vi "alternative instance of filter.vi"(7 "bandwidth":enum16{"20MHz", "40MHz"}(ring), 9 "input valid":bool, 10 "input cluster":T1) -> (1 "output valid":bool, 2 "sample out":T1)   [LabVIEW 2020]
uses:
  <vilib>/rvi/IPIntegrationNode/IPINode_Typedef/niFpgaIPINodeSupportedFamilies.ctl
  <vilib>/rvi/IPIntegrationNode/IPINode_Utilities/niFpgaIPINodeSimCore.vi
  <vilib>/rvi/XilinxIP/XIPIN_XNode/niFpgaXIPIN.xnode
  Untitled 3/FIR Compiler 3 1/xsim.dir/FIR_Compiler_3_1_CC812A82826341AB8BB5EFDFB4B49B09/xsimk_CC812A82826341AB8BB5EFDFB4B49B09.dll
  <vilib>/rvi/IPIntegrationNode/IPINode_Xnode/niFpgaIPINode.xnode
  Untitled 3/FIR Compiler 3 1 2/xsim.dir/FIR_Compiler_3_1_2_1438C8CDDF83493586378C164F746E96/xsimk_1438C8CDDF83493586378C164F746E96.dll
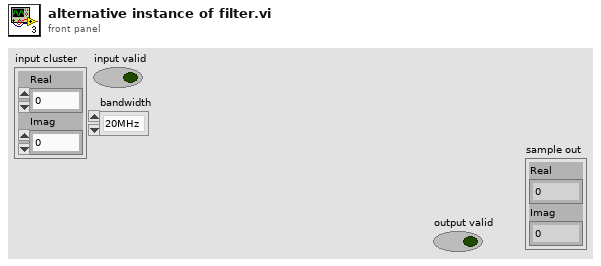
[diagram p1: front panel]
types:
  T1 = cluster{"Real":fxp<+/-,16,3>, "Imag":fxp<+/-,16,3>}
  T2 = typedef "niFpgaIPINodeSupportedFamilies.ctl" = cluster{"unlimited?":bool, "supported targets":string[]}
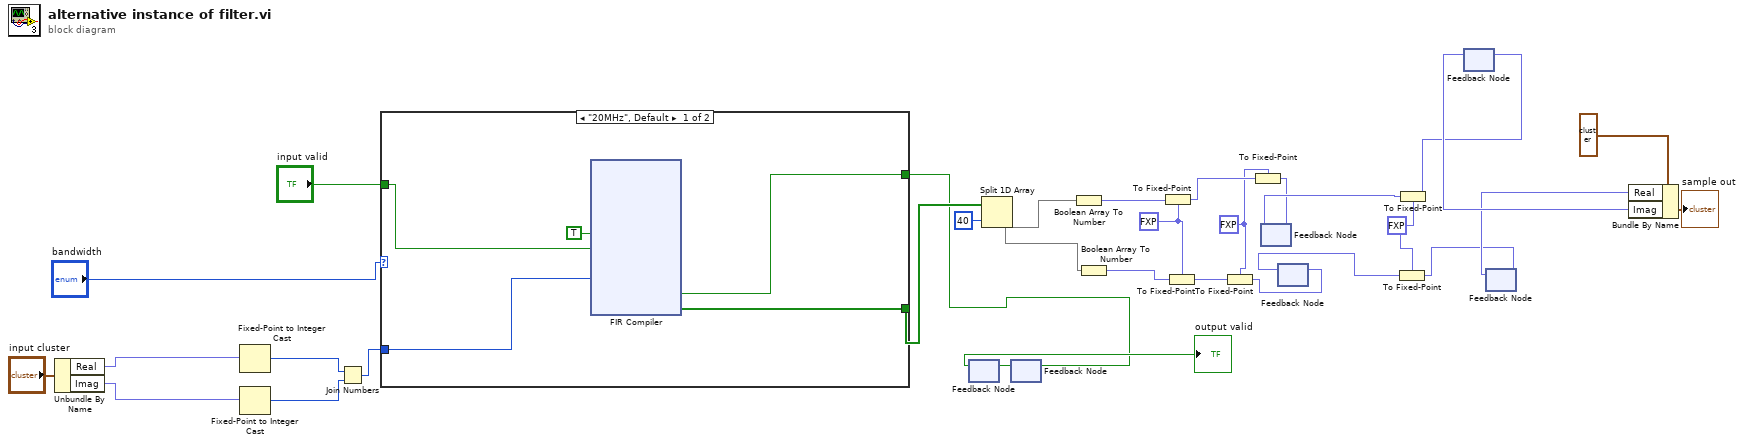
[diagram p0: block diagram]
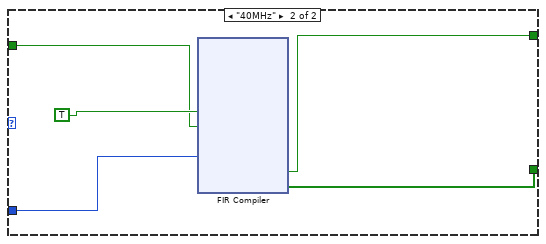
[diagram p2: hidden frame]
diagram:
  w10 = fxp<+/-,16,3> 0.0 ("fixed-point type")
  w9 = fxp<+/-,18,5> 0.0 ("fixed-point type")
  w8 = fxp<+/-,34,4> 0.0 ("fixed-point type")
  n1 = Unbundle By Name("input cluster") -> ("Real"=w12:fxp<+/-,16,3>, "Imag"=w13:fxp<+/-,16,3>)
  n2 = Fixed-Point to Integer Cast(1:w12) -> (0:w14:i16)
  n3 = Fixed-Point to Integer Cast(1:w13) -> (0:w15:i16)
  n4 = Join Numbers(hi=w14, lo=w15) -> ((hi.lo)=w17:u32)
  n5 = case shown="\"20MHz\", Default" "bandwidth" {
    tunnel: w17 -> [w37 w106]
    tunnel: [w36 w108] -> w30
    tunnel: [w35 w107] -> w1
    tunnel: "input valid" -> [w34 w104]
    frame "20MHz", Default {
      n6 = xnode ("FIR Compiler")("aclken"=TRUE, "s_axis_data_tvalid"=w34, "s_axis_data_tdata"=w37) -> ("m_axis_data_tvalid"=w35:bool, "m_axis_data_tdata"=w36:bool[])  [unwired: 1 out]
    }
    frame "40MHz" {
      n7 = xnode ("FIR Compiler")("aclken"=TRUE, "s_axis_data_tvalid"=w104, "s_axis_data_tdata"=w106) -> ("m_axis_data_tvalid"=w107:bool, "m_axis_data_tdata"=w108:bool[])  [unwired: 1 out]
    }
  }
  n8 = feedback #1() -> (→"output valid":bool)  [unwired: 1 in]
  n9 = Split 1D Array(array=w30, index=40) -> (first subarray=w19:bool[], second subarray=w20:bool[])
  n10 = feedback #2() -> (w2:bool)  [unwired: 1 in]
  n11 = feedback-in #1(w2) -> ()
  n12 = feedback-in #2(w1) -> ()
  n13 = Boolean Array To Number(Boolean array=w19) -> (number=w21:fxp<+/-,40,10>)
  n14 = Boolean Array To Number(Boolean array=w20) -> (number=w22:fxp<+/-,40,10>)
  n15 = To Fixed-Point(fixed-point type=w8, number=w21) -> (fixed-point=w23:fxp<+/-,34,4>)
  n16 = To Fixed-Point(fixed-point type=w8, number=w22) -> (fixed-point=w24:fxp<+/-,34,4>)
  n17 = To Fixed-Point(fixed-point type=w9, number=w24) -> (fixed-point=w4:fxp<+/-,18,5>)
  n18 = To Fixed-Point(fixed-point type=w9, number=w23) -> (fixed-point=w3:fxp<+/-,18,5>)
  n19 = feedback #3() -> (w28:fxp<+/-,18,5>)  [unwired: 1 in]
  n20 = feedback-in #3(w3) -> ()
  n21 = feedback #4() -> (w27:fxp<+/-,18,5>)  [unwired: 1 in]
  n22 = feedback-in #4(w4) -> ()
  n23 = To Fixed-Point(fixed-point type=w10, number=w27) -> (fixed-point=w6:fxp<+/-,16,3>)
  n24 = To Fixed-Point(fixed-point type=w10, number=w28) -> (fixed-point=w5:fxp<+/-,16,3>)
  n25 = feedback #5() -> (w26:fxp<+/-,16,3>)  [unwired: 1 in]
  n26 = feedback-in #5(w5) -> ()
  n27 = feedback #6() -> (w25:fxp<+/-,16,3>)  [unwired: 1 in]
  n28 = feedback-in #6(w6) -> ()
  n29 = Bundle By Name(cluster=T1 {"Real"=0.0, "Imag"=0.0} ("Complex"), "Real"=w25, "Imag"=w26) -> (→"sample out":T1)
